vi "libera.vi"() -> ()   [LabVIEW 2010]
uses:
  chaos-common-crest/LabVIEW/LV14/chaosui-crest/chaosui-crest.lvlib
  chaos-common-crest/LabVIEW/LV14/chaosui-crest/VIs/ChaosDevState.ctl
  <vilib>/Utility/file.llb/Write To Spreadsheet File (I64).vi
panel:
  out "DD2":cluster{"VA":i32, "VB":i32, "VC":i32, "VD":i32}(graph)
  out "SA":cluster{"VA":i32, "VB":i32, "VC":i32, "VD":i32}(graph)
  out "DD":cluster{i32[], i32[]}[](graph)
  in  "DataFile":path
  out "libera_error":i32
  out "STATUS":string
  out "SA_OUT":T1(array[cluster])
  out "ADC_CW":T2(array[cluster])
  out "AVG_OUT":cluster{"AVG":i32}[](array[cluster])
  out "ADC_SP":T3(array[cluster])
  in  "AVG":bool=TRUE
  in  "STATE":bool=TRUE
  in  "stop":bool
  in  "loops":i32=10
  in  "DECIMATED":bool
  out "DD_OUT":T4(array[cluster])
  in  "refresh (ms)":u32=200
  out "samples":i32
  out "mode":i32
  out "Device State":T5
  out "nok":i32
  out "dev_error":bool
  out "acquisitions":u64
  out "timestamp":u64
  in  "Samples":u32=10
  in  "TRIGGERED":bool
  in  "ADC CW":bool
  in  "ADC SP":bool
  in  "SA":bool
  in  "DD":bool
  in  "!CHAOS URL":string="chaost-webui1.chaos.lnf.infn.it:8081"
  in  "LiberaID":string="LIBERA02/LIBERA_ACQUIRE0"
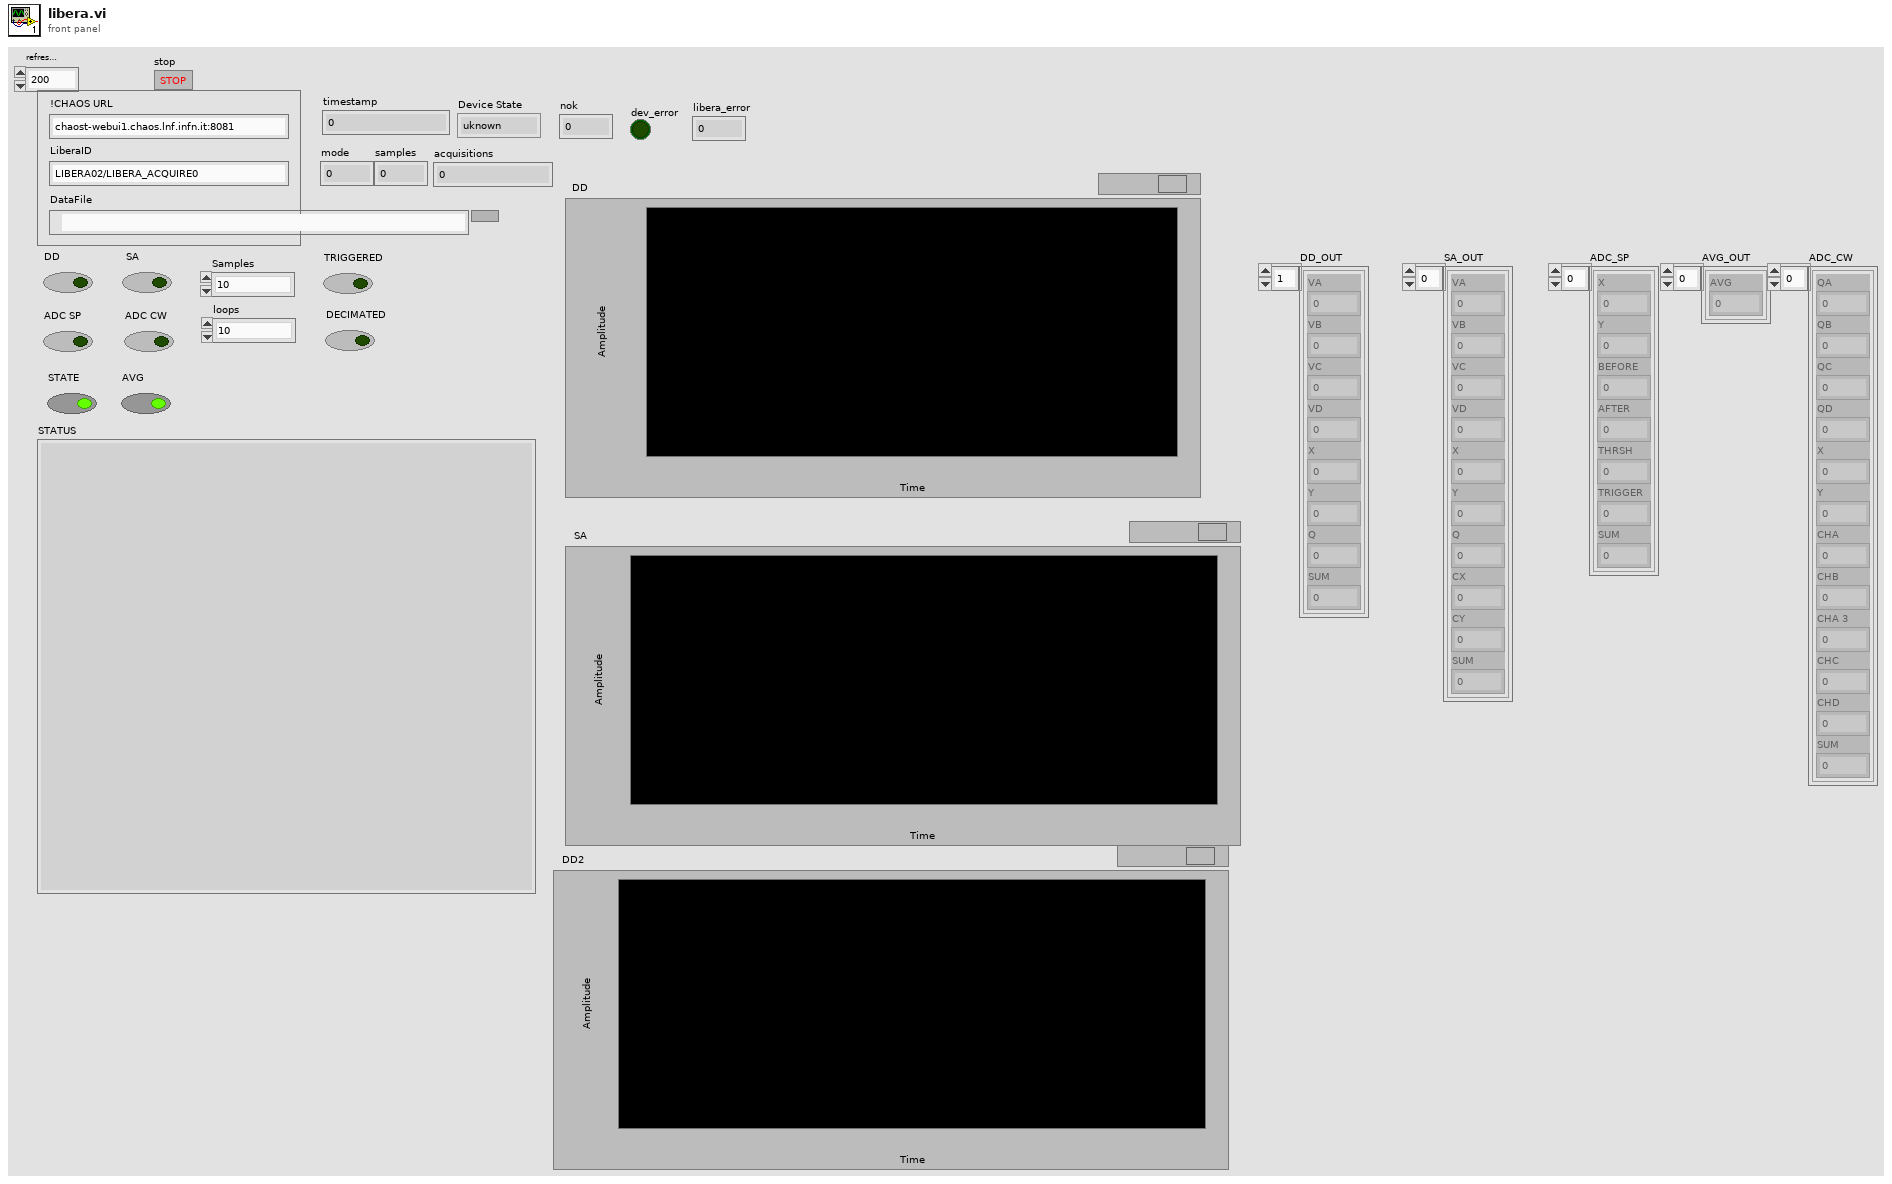
[diagram p1: front panel]
types:
  T1 = cluster{"VA":i32, "VB":i32, "VC":i32, "VD":i32, "X":i32, "Y ":i32, "Q":i32, "CX":i32, "CY":i32, "SUM":i32}[]
  T2 = cluster{"QA":i32, "QB":i32, "QC":i32, "QD":i32, "X":i32, "Y":i32, "CHA":i32, "CHB":i32, "CHA 3":i32, "CHC":i32, "CHD":i32, "SUM":i32}[]
  T3 = cluster{"X":i32, "Y":i32, "BEFORE":i32, "AFTER":i32, "THRSH":i32, "TRIGGER":i32, "SUM":i32}[]
  T4 = cluster{"VA":i32, "VB":i32, "VC":i32, "VD":i32, "X":i32, "Y ":i32, "Q":i32, "SUM":i32}[]
  T5 = typedef "ChaosDevState.ctl" = enum16{"uknown", "stop", "init", "deinit", "start"}
  T6 = typedef "LabVIEWHTTPClient.lvlib/ClientHandle.ctl" = refnum<k1>
  T7 = cluster{"client handle out":T6, "chaoswanurl":string}
  T8 = enum16{"stopAcquire", "setTime", "acquireAVG", "acquireADCSP", "acquireADCCW", "acquireStream", "acquireDD"}
  T9 = cluster{"VA":i32, "VB":i32, "VC":i32, "VD":i32, "X":i32, "Y ":i32, "Q":i32, "CX":i32, "CY":i32, "SUM":i32}
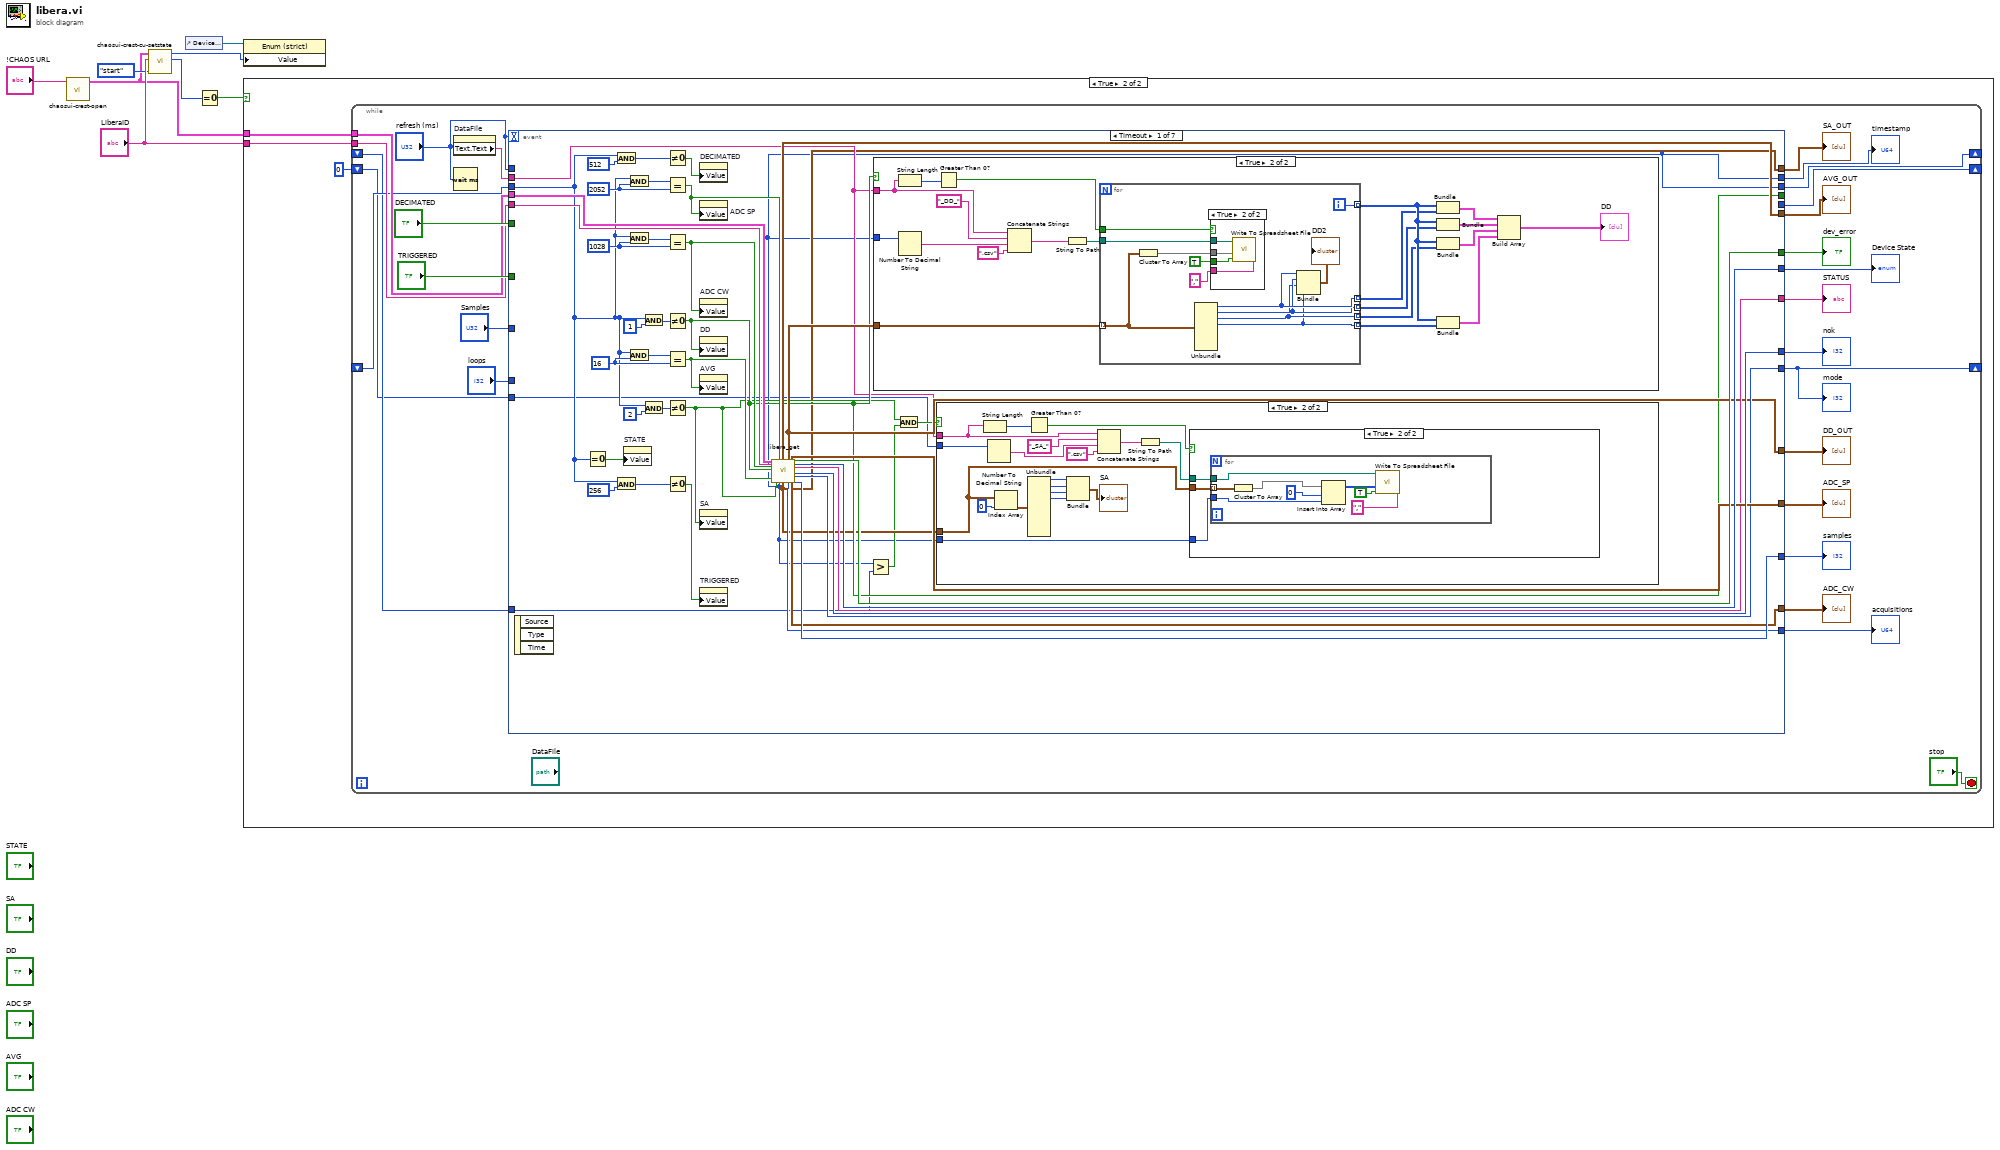
[diagram p0: block diagram]
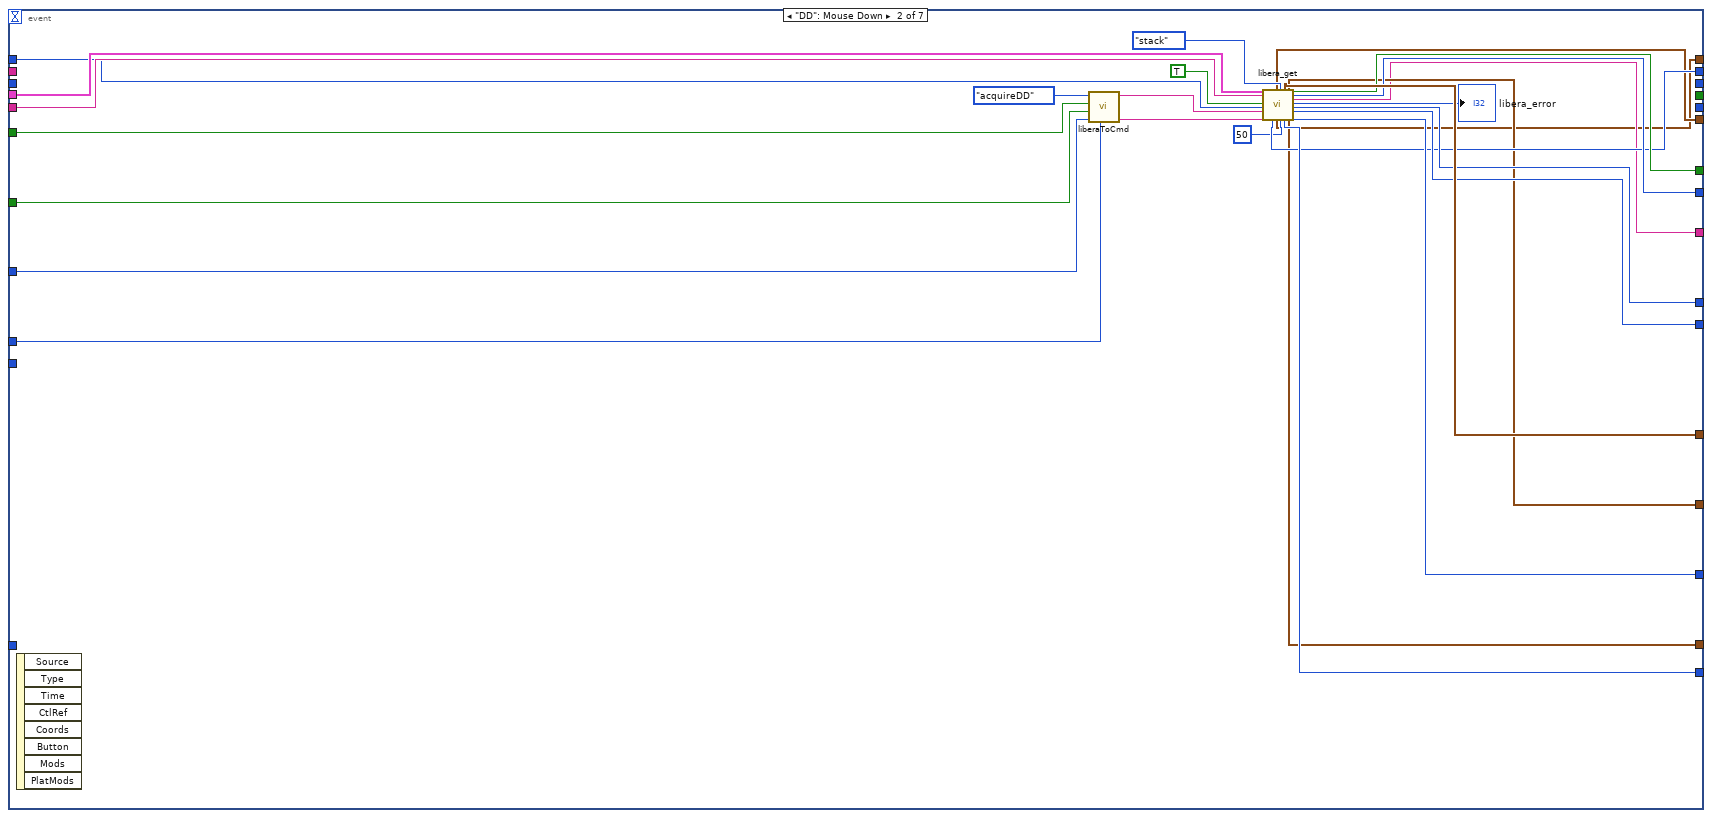
[diagram p7: hidden frame]
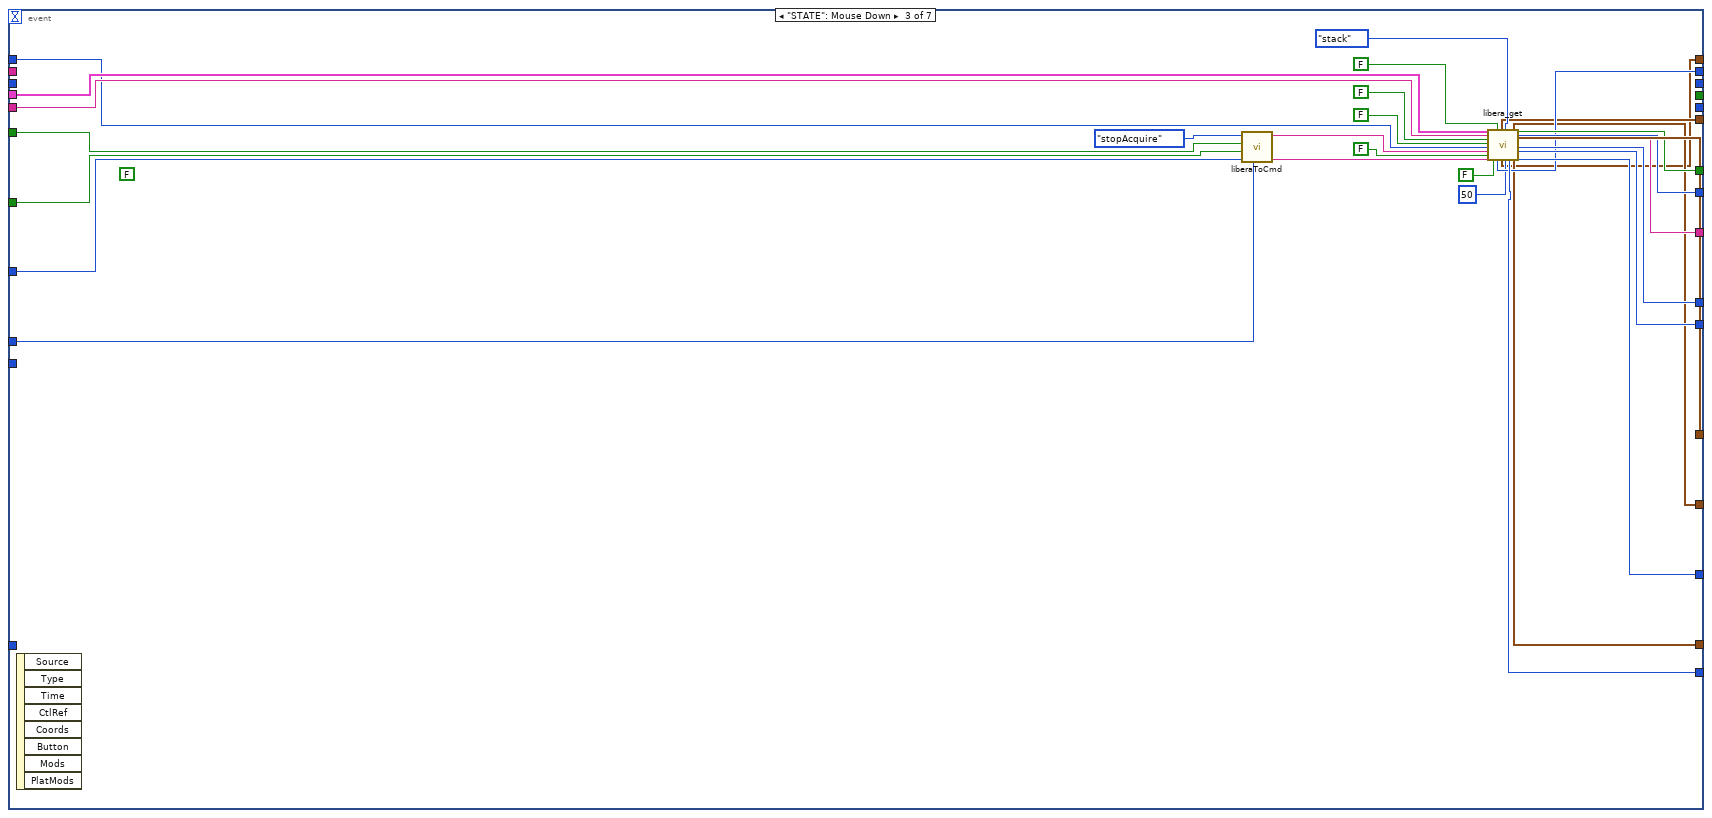
[diagram p8: hidden frame]
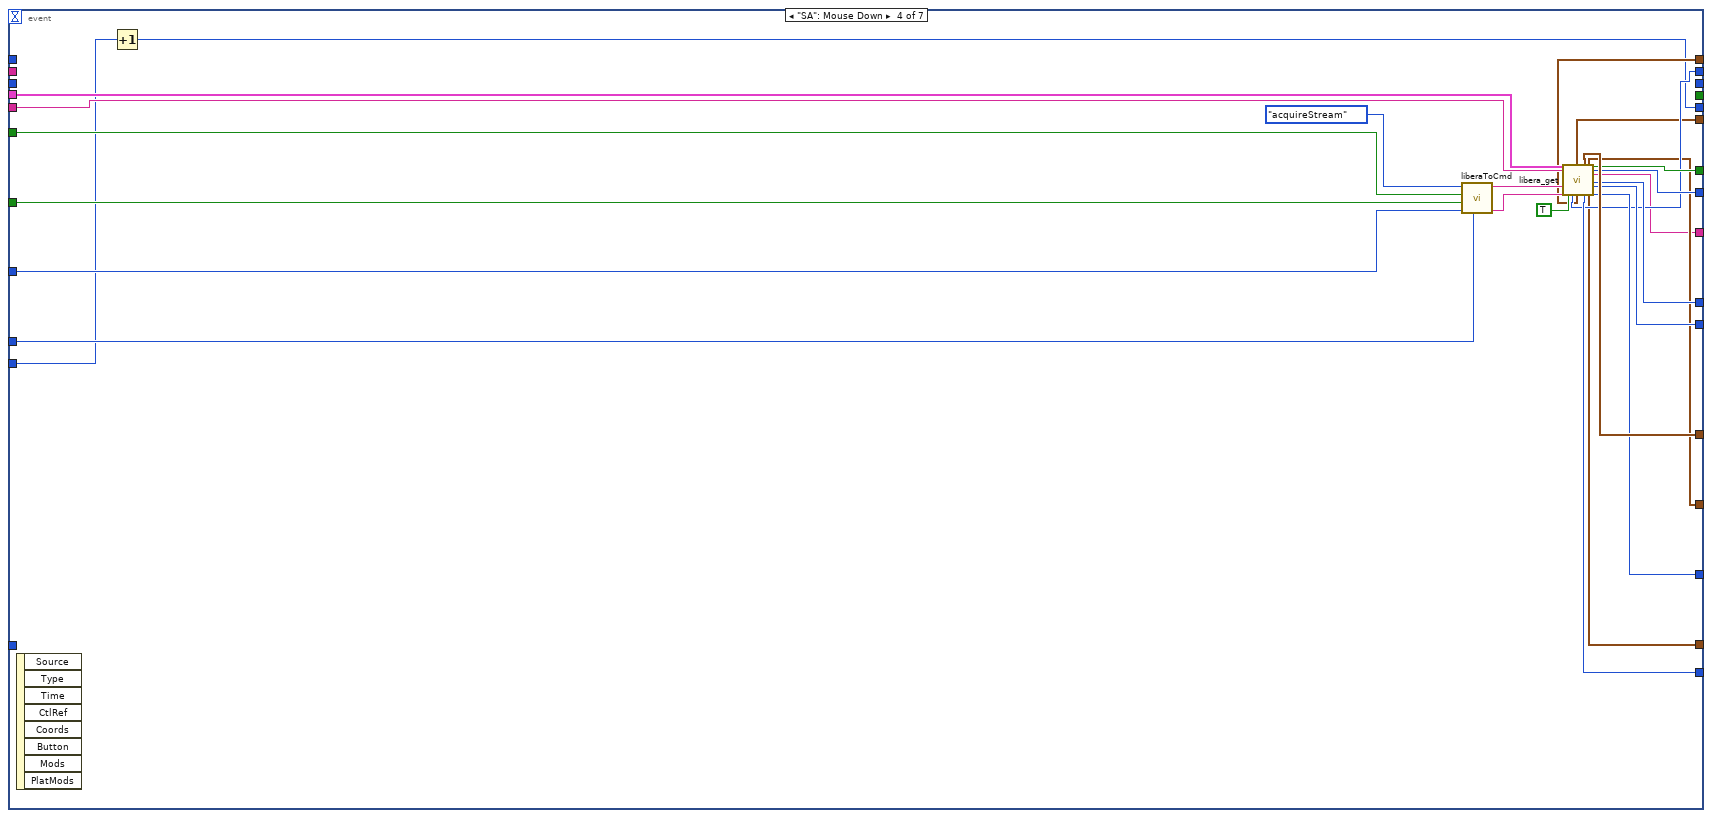
[diagram p9: hidden frame]
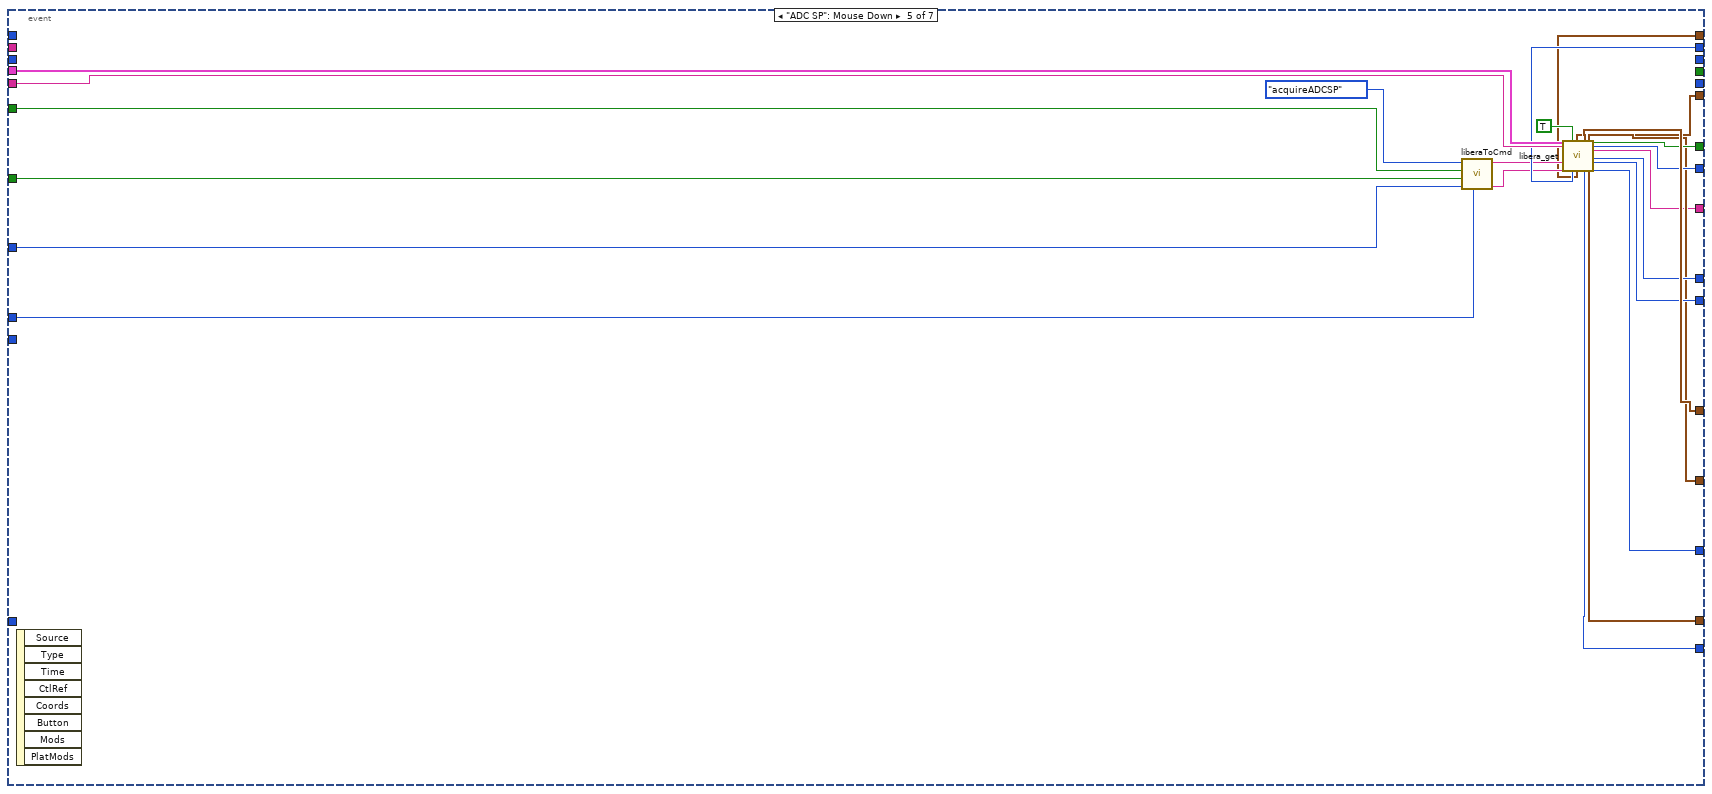
[diagram p10: hidden frame]
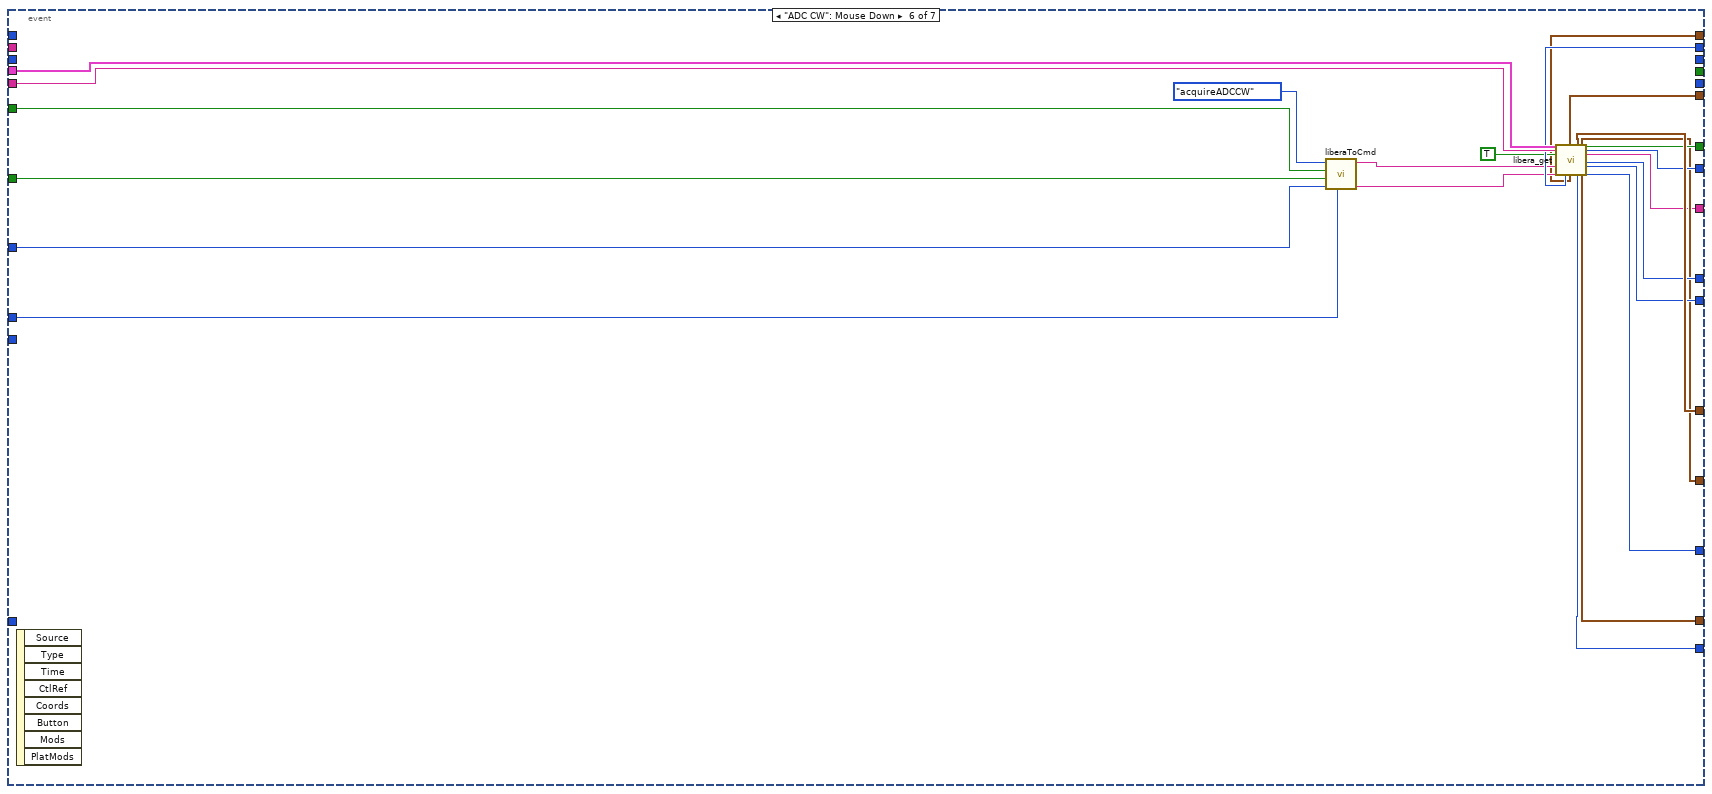
[diagram p11: hidden frame]
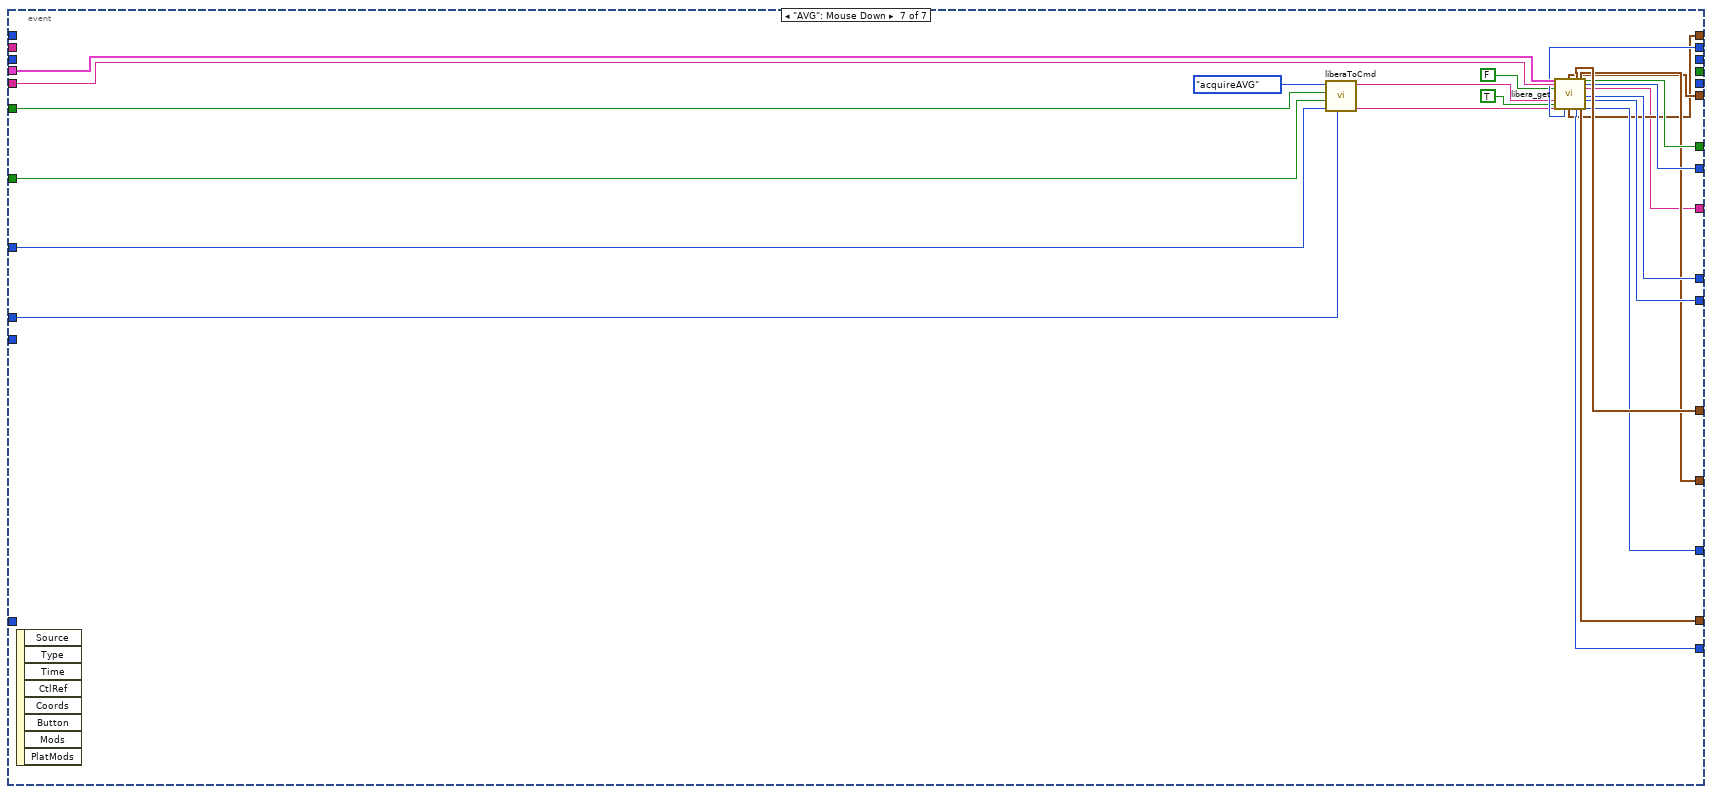
[diagram p12: hidden frame]
diagram:
  n1 = call "chaosui-crest-open.vi"("chaoswanurl"="!CHAOS URL") -> ("handle"=w1:T7)  [unwired: 10 in]
  n2 = call "chaosui-crest-cu-setstate.vi"("dev_state"=ChaosDevState."start", "cuname"="LiberaID", "handleConnection"=w1) -> ("nok"=w3:i32, "dev_state_out"=w4:T5)  [unwired: 1 in, 3 out]
  n3 = control-ref of="Device State"() -> (w5:refnum<vi>)
  n4 = Equal To 0?(x=w3) -> (x = 0?=w7:bool)
  n5 = property class="Enum (strict)"(reference=w5, "Value"=w4) -> ()  [unwired: 1 in, 2 out]
  n6 = case shown="True" w7 {
    tunnel: w1 -> [_ w11]
    tunnel: "LiberaID" -> [_ w10]
    frame False {
    }
    frame True {
      n7 = while {
        tunnel: w11 -> [w27]
        tunnel: w10 -> [w26]
        shift-right: [w25] -> _
        shift-left: _ -> [w24]
        shift-right: [w15] -> _
        shift-left: _ -> [w14]
        shift-right: [w12] -> _
        shift-left: 0 -> [w13]
        stop <- "stop" stop-if-true
        n8 = property on="DataFile" class="Path"() -> ("Text.Text"=w16:string)  [unwired: 2 in, 2 out]
        n9 = Wait (ms)(milliseconds to wait="refresh (ms)") -> ()  [unwired: 1 out]
        n10 = event shown="[0] Timeout" {
          selector: _ -> [_ _ _ _ _ _ _]
          dyn-events: _ -> [_ _ _ _ _ _ _]
          timeout: "refresh (ms)" -> [_ _ _ _ _ _ _]
          tunnel: w27 -> [w81 w173 w203 w228 w251 w274 w298]
          tunnel: w26 -> [w80 w172 w202 w227 w250 w273 w297]
          tunnel: [w79 w170 w200 w225 w248 w271 w295] -> w38
          tunnel: [w78 w169 w199 w224 w247 w270 w294] -> w37
          tunnel: [w77 w168 w198 w223 w246 w269 w293] -> w36
          tunnel: [w49 w167 w197 w222 w245 w268 w292] -> w25
          tunnel: [w76 w166 w196 w221 w244 w267 w291] -> w35
          tunnel: [w75 w165 w195 w220 w243 w266 w290] -> w34
          tunnel: [w40 w164 w194 w219 w242 w265 w289] -> w17
          tunnel: [w48 w171 w201 w226 w249 w272 w296] -> w18
          tunnel: "Samples" -> [_ w163 w193 w218 w241 w264 w288]
          tunnel: "TRIGGERED" -> [_ w162 w192 w217 w240 w263 w287]
          tunnel: "DECIMATED" -> [_ w161 w191 w216 w239 w262 w286]
          tunnel: "loops" -> [_ w158 w188 w212 w235 w258 w282]
          tunnel: "refresh (ms)" -> [_ w156 w186 _ _ _ _]
          tunnel: w24 -> [w55 _ _ _ _ _ _]
          tunnel: [w52 w152 w177 w210 w233 w256 w279] -> w23
          tunnel: [w50 w151 w176 w209 w232 w255 w278] -> w22
          tunnel: [w53 w149 w175 w206 w230 w253 w277] -> w21
          tunnel: [w44 w148 w174 w207 w229 w252 w276] -> w20
          tunnel: [w51 w150 w178 w208 w231 w254 w275] -> w19
          tunnel: [w47 _ _ _ _ _ _] -> _
          tunnel: w16 -> [w46 _ _ _ _ _ _]
          tunnel: [w40 _ _ _ _ _ _] -> w15
          tunnel: w14 -> [w43 _ _ _ _ _ _]
          tunnel: w13 -> [w39 _ _ w205 _ _ _]
          tunnel: [_ _ _ w204 _ _ _] -> w12
          event Timeout {
            w62 = u32 16 ("y")
            w66 = u32 1028 ("y")
            w68 = u32 2052 ("y")
            n11 = event-data() -> ()  [unwired: 1 in, 3 out]
            n12 = Equal To 0?(x=w55) -> (x = 0?=w72:bool)
            n13 = And(x=w55, y=u32 512) -> (x .and. y?=w56:u32)
            n14 = And(x=w55, y=u32 256) -> (x .and. y?=w60:u32)
            n15 = property on="STATE" class="Bool (strict)"("Value"=w72) -> ()  [unwired: 2 in, 2 out]
            n16 = And(x=w55, y=w68) -> (x .and. y?=w69:u32)
            n17 = And(x=w55, y=w66) -> (x .and. y?=w65:u32)
            n18 = And(x=w55, y=w62) -> (x .and. y?=w63:u32)
            n19 = And(x=w55, y=u32 1) -> (x .and. y?=w73:u32)
            n20 = And(x=w55, y=u32 2) -> (x .and. y?=w70:u32)
            n21 = Not Equal To 0?(x=w56) -> (x != 0?=w54:bool)
            n22 = Equal?(x=w69, y=w68) -> (x = y?=w67:bool)
            n23 = Equal?(x=w65, y=w66) -> (x = y?=w64:bool)
            n24 = Not Equal To 0?(x=w73) -> (x != 0?=w47:bool)
            n25 = Equal?(x=w63, y=w62) -> (x = y?=w61:bool)
            n26 = Not Equal To 0?(x=w70) -> (x != 0?=w45:bool)
            n27 = Not Equal To 0?(x=w60) -> (x != 0?=w58:bool)
            n28 = property on="DECIMATED" class="Bool (strict)"("Value"=w54) -> ()  [unwired: 2 in, 2 out]
            n29 = property on="ADC SP" class="Bool (strict)"("Value"=w67) -> ()  [unwired: 2 in, 2 out]
            n30 = property on="ADC CW" class="Bool (strict)"("Value"=w64) -> ()  [unwired: 2 in, 2 out]
            n31 = property on="DD" class="Bool (strict)"("Value"=w47) -> ()  [unwired: 2 in, 2 out]
            n32 = property on="AVG" class="Bool (strict)"("Value"=w61) -> ()  [unwired: 2 in, 2 out]
            n33 = property on="SA" class="Bool (strict)"("Value"=w45) -> ()  [unwired: 2 in, 2 out]
            n34 = property on="TRIGGERED" class="Bool (strict)"("Value"=w58) -> ()  [unwired: 2 in, 2 out]
            n35 = call "libera_get.vi"("handleConnection"=w81, "cuname"=w80, "Enable ADC CW"=w64, "Enable DD"=w47, "Enable AVG"=w61, "Enable SA"=w45, "Enable ADC SP"=w67) -> ("timestamp"=w40:u64, "AVG"=w50:cluster{"AVG":i32}[], "SA"=w44:T1, "DD"=w48:T4, "acquisitions"=w75:u64, "ADC_SP"=w52:T3, "ADC_CW"=w53:T2, "dev_error"=w79:bool, "dev_state"=w78:T5, "STATUS"=w51:string, "nok"=w77:i32, "mode"=w49:i32, "samples"=w76:i32)  [unwired: 7 in, 1 out]
            n36 = Greater?(x=w40, y=w43) -> (0:w41:bool)
            n37 = case shown="True" w47 {
              tunnel: w40 -> [_ w130]
              tunnel: w48 -> [_ w124]
              tunnel: w46 -> [_ w116]
              frame False {
              }
              frame True {
                n38 = String Length(string=w116) -> (length=w117:i32)
                n39 = Number To Decimal String(number=w130) -> (decimal integer string=w129:string)  [unwired: 1 in]
                n40 = Greater Than 0?(x=w117) -> (x > 0?=w115:bool)
                n41 = Concatenate Strings(w116, "_DD_" ("string"), w129, ".csv" ("name or relative path")) -> (w126:string)
                n42 = String To Path(string=w126) -> (path=w125:path)
                n43 = for {
                  tunnel: w125 -> [w142]
                  tunnel: w124 -> [w138] mode=indexing
                  tunnel: [w135] -> w111 mode=indexing
                  tunnel: [w137] -> w123 mode=indexing
                  tunnel: [w134] -> w114 mode=indexing
                  tunnel: [w133] -> w113 mode=indexing
                  tunnel: [w132] -> w112 mode=indexing
                  tunnel: w115 -> [w136]
                  i -> [w137]
                  n44 = Cluster To Array(cluster=w138) -> (array=w141:i32[])
                  n45 = Unbundle(w138) -> ("VA"=w135:i32, "VB"=w134:i32, "VC"=w133:i32, "VD"=w132:i32)  [unwired: 4 out]
                  n46 = case shown="True" w136 {
                    tunnel: w142 -> [_ w146]
                    tunnel: w141 -> [_ w145]
                    tunnel: TRUE ("append to file? (new file:F)") -> [_ w144]
                    tunnel: "," ("delimiter (\\t)") -> [_ w143]
                    frame False {
                    }
                    frame True {
                      n47 = call-poly <vilib>:"Write To Spreadsheet File.vi"("delimiter (\\t)"=w143, "append to file? (new file:F)"=w144, "1D data"=w145, "file path (dialog if empty)"=w146) -> ()  [unwired: 4 in, 1 out]
                    }
                  }
                  n48 = Bundle("VA"=w135, "VB"=w134, "VC"=w133, "VD"=w132) -> (→"DD2":cluster{"VA":i32, "VB":i32, "VC":i32, "VD":i32})  [unwired: 1 in]
                }
                n49 = Bundle(w123, w111) -> (w122:cluster{i32[], i32[]})  [unwired: 1 in]
                n50 = Bundle(w123, w114) -> (w121:cluster{i32[], i32[]})  [unwired: 1 in]
                n51 = Bundle(w123, w113) -> (w120:cluster{i32[], i32[]})  [unwired: 1 in]
                n52 = Bundle(w123, w112) -> (w119:cluster{i32[], i32[]})  [unwired: 1 in]
                n53 = Build Array(w122, w121, w120, w119) -> (→"DD":cluster{i32[], i32[]}[])
              }
            }
            n54 = And(x=w45, y=w41) -> (x .and. y?=w42:bool)
            n55 = case shown="True" w42 {
              tunnel: w44 -> [_ w94]
              tunnel: w46 -> [_ w87]
              tunnel: w40 -> [_ w91]
              tunnel: w39 -> [_ w96]
              frame False {
              }
              frame True {
                n56 = String Length(string=w87) -> (length=w88:i32)
                n57 = Number To Decimal String(number=w96) -> (decimal integer string=w95:string)  [unwired: 1 in]
                n58 = Index Array(array=w94, index=0) -> (element=w92:T9)
                n59 = Greater Than 0?(x=w88) -> (x > 0?=w89:bool)
                n60 = Unbundle(w92) -> ("VA"=w86:i32, "VB"=w85:i32, "VC"=w84:i32, "VD"=w83:i32)  [unwired: 6 out]
                n61 = Bundle("VA"=w86, "VB"=w85, "VC"=w84, "VD"=w83) -> (→"SA":cluster{"VA":i32, "VB":i32, "VC":i32, "VD":i32})  [unwired: 1 in]
                n62 = Concatenate Strings(w87, "_SA_" ("string"), w95, ".csv" ("name or relative path")) -> (w98:string)
                n63 = String To Path(string=w98) -> (path=w97:path)
                n64 = case shown="True" w89 {
                  tunnel: w97 -> [_ w102]
                  tunnel: w94 -> [_ w101]
                  tunnel: w91 -> [_ w100]
                  frame False {
                  }
                  frame True {
                    n65 = for {
                      tunnel: w102 -> [w110]
                      tunnel: w101 -> [w109] mode=indexing
                      tunnel: w100 -> [w104]
                      n66 = Cluster To Array(cluster=w109) -> (array=w106:i32[])
                      n67 = Insert Into Array(array=w106, index=0, new element=w104) -> (w103:i32[])
                      n68 = call-poly <vilib>:"Write To Spreadsheet File.vi"("delimiter (\\t)"="," ("delimiter (\\t)"), "append to file? (new file:F)"=TRUE, "1D data"=w103, "file path (dialog if empty)"=w110) -> ()  [unwired: 4 in, 1 out]
                    }
                  }
                }
              }
            }
          }
          event "DD": Mouse Down {
            n69 = event-data() -> ()  [unwired: 1 in, 8 out]
            n70 = call "liberaToCmd.vi"("loops"=w158, "samples"=w163, "triggered"=w162, "decimated"=w161, "cmd"=T8."acquireDD") -> ("jsonargs"=w159:string, "cmd"=w160:string)  [unwired: 5 in]
            n71 = call "libera_get.vi"("handleConnection"=w173, "cuname"=w172, "Enable DD"=TRUE, "sched (ms)"=w156, "cmd"=w160, "args"=w159, "cmd submission mode"=enum16{"stack", "kill previous"}."stack", "prio"=50) -> ("timestamp"=w164:u64, "AVG"=w151:cluster{"AVG":i32}[], "SA"=w148:T1, "DD"=w171:T4, "acquisitions"=w165:u64, "ADC_SP"=w152:T3, "ADC_CW"=w149:T2, "dev_error"=w170:bool, "dev_state"=w169:T5, "STATUS"=w150:string, "libera_error"=→"libera_error":i32, "nok"=w168:i32, "mode"=w167:i32, "samples"=w166:i32)  [unwired: 6 in]
          }
          event "STATE": Mouse Down {
            (unwired) FALSE ("Enable SA")
            n72 = event-data() -> ()  [unwired: 1 in, 8 out]
            n73 = call "liberaToCmd.vi"("loops"=w188, "samples"=w193, "triggered"=w192, "decimated"=w191, "cmd"=T8."stopAcquire") -> ("jsonargs"=w189:string, "cmd"=w190:string)  [unwired: 5 in]
            n74 = call "libera_get.vi"("handleConnection"=w203, "cuname"=w202, "Enable ADC CW"=FALSE, "Enable DD"=FALSE, "sched (ms)"=w186, "cmd"=w190, "Enable AVG"=FALSE, "args"=w189, "Enable SA"=FALSE, "Enable ADC SP"=FALSE, "cmd submission mode"=enum16{"stack", "kill previous"}."stack", "prio"=50) -> ("timestamp"=w194:u64, "AVG"=w176:cluster{"AVG":i32}[], "SA"=w174:T1, "DD"=w201:T4, "acquisitions"=w195:u64, "ADC_SP"=w177:T3, "ADC_CW"=w175:T2, "dev_error"=w200:bool, "dev_state"=w199:T5, "STATUS"=w178:string, "nok"=w198:i32, "mode"=w197:i32, "samples"=w196:i32)  [unwired: 2 in, 1 out]
          }
          event "SA": Mouse Down {
            n75 = event-data() -> ()  [unwired: 1 in, 8 out]
            n76 = Increment(x=w205) -> (x+1=w204:i32)
            n77 = call "liberaToCmd.vi"("loops"=w212, "samples"=w218, "triggered"=w217, "decimated"=w216, "cmd"=T8."acquireStream") -> ("jsonargs"=w213:string, "cmd"=w214:string)  [unwired: 5 in]
            n78 = call "libera_get.vi"("handleConnection"=w228, "cuname"=w227, "cmd"=w214, "args"=w213, "Enable SA"=TRUE) -> ("timestamp"=w219:u64, "AVG"=w209:cluster{"AVG":i32}[], "SA"=w207:T1, "DD"=w226:T4, "acquisitions"=w220:u64, "ADC_SP"=w210:T3, "ADC_CW"=w206:T2, "dev_error"=w225:bool, "dev_state"=w224:T5, "STATUS"=w208:string, "nok"=w223:i32, "mode"=w222:i32, "samples"=w221:i32)  [unwired: 9 in, 1 out]
          }
          event "ADC SP": Mouse Down {
            n79 = event-data() -> ()  [unwired: 1 in, 8 out]
            n80 = call "liberaToCmd.vi"("loops"=w235, "samples"=w241, "triggered"=w240, "decimated"=w239, "cmd"=T8."acquireADCSP") -> ("jsonargs"=w236:string, "cmd"=w237:string)  [unwired: 5 in]
            n81 = call "libera_get.vi"("handleConnection"=w251, "cuname"=w250, "cmd"=w237, "args"=w236, "Enable ADC SP"=TRUE) -> ("timestamp"=w242:u64, "AVG"=w232:cluster{"AVG":i32}[], "SA"=w229:T1, "DD"=w249:T4, "acquisitions"=w243:u64, "ADC_SP"=w233:T3, "ADC_CW"=w230:T2, "dev_error"=w248:bool, "dev_state"=w247:T5, "STATUS"=w231:string, "nok"=w246:i32, "mode"=w245:i32, "samples"=w244:i32)  [unwired: 9 in, 1 out]
          }
          event "ADC CW": Mouse Down {
            n82 = event-data() -> ()  [unwired: 1 in, 8 out]
            n83 = call "liberaToCmd.vi"("loops"=w258, "samples"=w264, "triggered"=w263, "decimated"=w262, "cmd"=T8."acquireADCCW") -> ("jsonargs"=w259:string, "cmd"=w260:string)  [unwired: 5 in]
            n84 = call "libera_get.vi"("handleConnection"=w274, "cuname"=w273, "Enable ADC CW"=TRUE, "cmd"=w260, "args"=w259) -> ("timestamp"=w265:u64, "AVG"=w255:cluster{"AVG":i32}[], "SA"=w252:T1, "DD"=w272:T4, "acquisitions"=w266:u64, "ADC_SP"=w256:T3, "ADC_CW"=w253:T2, "dev_error"=w271:bool, "dev_state"=w270:T5, "STATUS"=w254:string, "nok"=w269:i32, "mode"=w268:i32, "samples"=w267:i32)  [unwired: 9 in, 1 out]
          }
          event "AVG": Mouse Down {
            n85 = event-data() -> ()  [unwired: 1 in, 8 out]
            n86 = call "liberaToCmd.vi"("loops"=w282, "samples"=w288, "triggered"=w287, "decimated"=w286, "cmd"=T8."acquireAVG") -> ("jsonargs"=w283:string, "cmd"=w284:string)  [unwired: 5 in]
            n87 = call "libera_get.vi"("handleConnection"=w298, "cuname"=w297, "Enable ADC CW"=FALSE, "cmd"=w284, "Enable AVG"=TRUE, "args"=w283) -> ("timestamp"=w289:u64, "AVG"=w278:cluster{"AVG":i32}[], "SA"=w276:T1, "DD"=w296:T4, "acquisitions"=w290:u64, "ADC_SP"=w279:T3, "ADC_CW"=w277:T2, "dev_error"=w295:bool, "dev_state"=w294:T5, "STATUS"=w275:string, "nok"=w293:i32, "mode"=w292:i32, "samples"=w291:i32)  [unwired: 8 in, 1 out]
          }
        }
        "timestamp" <- w17
        "acquisitions" <- w34
        "dev_error" <- w38
        "nok" <- w36
        "Device State" <- w37
        "mode" <- w25
        "samples" <- w35
        "DD_OUT" <- w18
        "ADC_SP" <- w23
        "AVG_OUT" <- w22
        "ADC_CW" <- w21
        "SA_OUT" <- w20
        "STATUS" <- w19
      }
    }
  }
